vi "Write Low Cutoff Freq.vi"(8 "error in (no error)":errorcluster, 10 "Low Cutoff Freq(Hz)":dbl, 11 "DataFilter in":refnum<class "DataFilter.lvclass">) -> (0 "error out":errorcluster, 3 "DataFilter out":refnum<class "DataFilter.lvclass">)   [LabVIEW 2010, in "DataFilter.lvclass"]
uses:
  DataFilter.lvclass
  DataFilter.lvclass/DataFilter.ctl
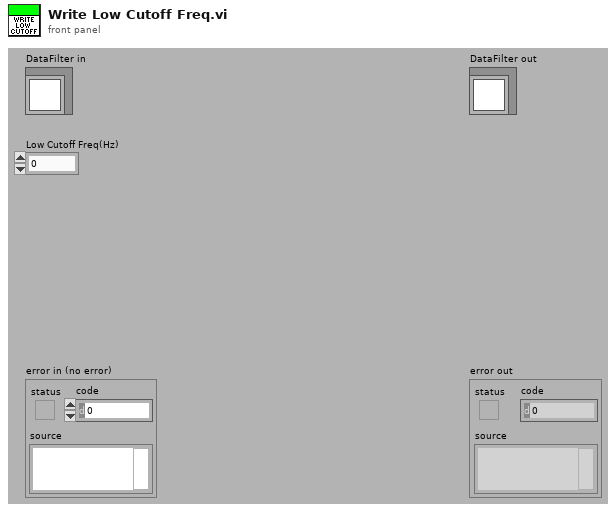
[diagram p1: front panel]
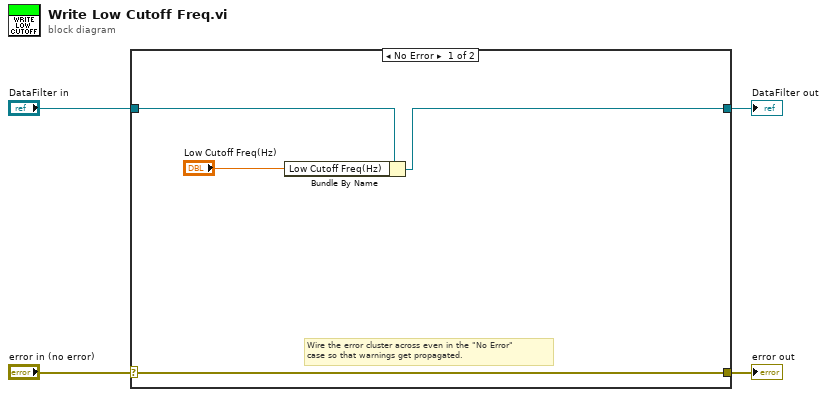
[diagram p0: block diagram]
diagram:
  n1 = case shown="No Error" "error in (no error)" {
    selector: "error in (no error)" -> [w8 w10]
    tunnel: [w8 w10] -> w3
    tunnel: [w6 w9] -> w1
    tunnel: "DataFilter in" -> [w7 w9]
    frame No Error {
      # "Wire the error cluster across even in the \"No Error\"\ncase so that warnings get propagated."
      n2 = Bundle By Name(cluster=w7, "Low Cutoff Freq(Hz)"="Low Cutoff Freq(Hz)") -> (w6:refnum<class "DataFilter.lvclass">)
    }
    frame Error {
    }
  }
  "error out" <- w3
  "DataFilter out" <- w1
